vi "Create from SCP Send.vi"(4 "Permissions":T1={"Owner"={"Read"=TRUE, "Write"=TRUE, "Execute"=FALSE}, "Group"={"Read"=TRUE, "Write"=FALSE, "Execute"=FALSE}, "Others"={"Read"=TRUE, "Write"=FALSE, "Execute"=FALSE}}, 8 "Error In":errorcluster, 9 "File Size":i64, 10 "Remote Destination Path":string, 11 "Session":refnum<class "Session.lvclass">) -> (0 "Error Out":errorcluster, 3 "Channel":refnum<class "Channel.lvclass">)   [LabVIEW 2018, in "Toolkit.lvlib" / "Channel.lvclass"]
uses:
  Channel.lvclass
  Session/Session.lvclass
  Type Definitions/Permissions.ctl
  Type Definitions/Modes.ctl
  Session/Session.lvclass/Session.ctl
  SSH/SSH.lvclass/SSH.ctl
  Channel.lvclass/Channel.ctl
  Toolkit.lvlib
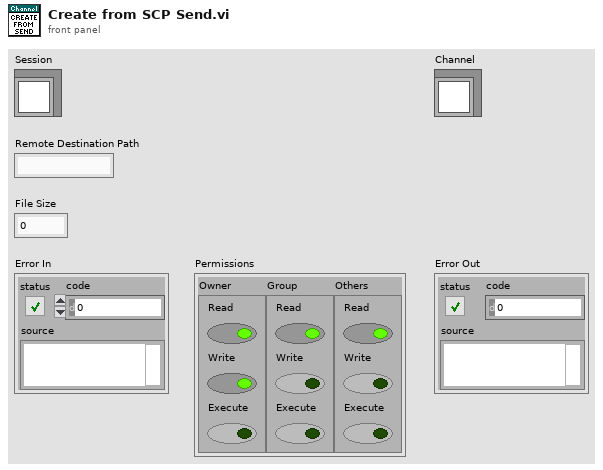
[diagram p1: front panel]
types:
  T1 = typedef "Toolkit.lvlib/Permissions.ctl" = cluster{"Owner":T2, "Group":T2, "Others":T2}
  T2 = typedef "Toolkit.lvlib/Modes.ctl" = cluster{"Read":bool, "Write":bool, "Execute":bool}
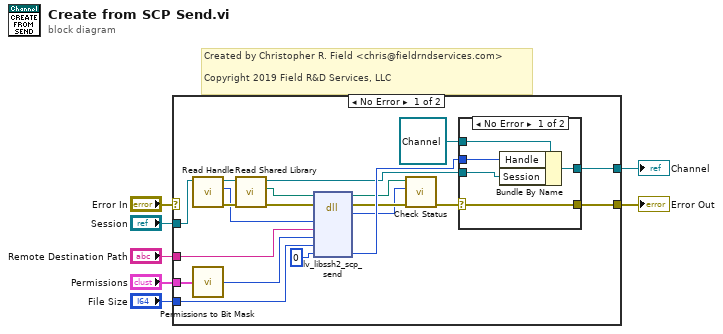
[diagram p0: block diagram]
diagram:
  # "Created by Christopher R. Field <chris@fieldrndservices.com>\n\nCopyright 2019 Field R&D Services, LLC"
  n1 = case shown="No Error" "Error In" {
    selector: "Error In" -> [_ w35]
    tunnel: [w25 w35] -> w6
    tunnel: "Session" -> [w26 _]
    tunnel: [w27 _] -> w4
    tunnel: "Permissions" -> [w23 _]
    tunnel: "Remote Destination Path" -> [w9 _]
    tunnel: "File Size" -> [w8 _]
    frame No Error {
      n2 = call "Read Handle.vi"("Session In"=w26) -> ("Erorr Out"=w21:errorcluster, "Handle"=w18:u64, "Session Out"=w22:refnum<class "Session.lvclass">)  [unwired: 8 in]
      n3 = call "Permissions to Bit Mask.vi"("Permissions"=w23) -> ("Bit Mask"=w10:u32)
      n4 = call "Read Shared Library.vi"("Error In"=w21, "Session In"=w22) -> ("Erorr Out"=w20:errorcluster, "libssh2lv Shared Library"=w19:path, "Session Out"=w11:refnum<class "Session.lvclass">)  [unwired: 7 in]
      n5 = dll-call lib="libssh2lv.*" fn="lv_libssh2_scp_send"(path in=w19, error in=w20, "session"=w18, "path"=w9, "mode"=w10, "file_size"=w8, "handle"=u64 0) -> (path out=w13:path, error out=w15:errorcluster, "status"=w14:i32, "handle"=w16:u64)  [unwired: 5 in]
      n6 = call "Check Status.vi"("Error In"=w15, "Status"=w14, "lv-libssh2 Shared Library In"=w13) -> ("Error Out"=w12:errorcluster)  [unwired: 7 in, 1 out]
      n7 = case shown="No Error" w12 {
        selector: w12 -> [w31 w34]
        tunnel: [w28 w33] -> w27
        tunnel: w16 -> [w32 _]
        tunnel: [w31 w34] -> w25
        tunnel: w11 -> [w30 _]
        tunnel: refnum<class "Channel.lvclass"> refnum ("Toolkit.lvlib:Channel.lvclass") -> [w29 w33]
        frame No Error {
          n8 = Bundle By Name(cluster=w29, "Handle"=w32, "Session"=w30) -> (w28:refnum<class "Channel.lvclass">)
        }
        frame Error {
        }
      }
    }
    frame Error {
    }
  }
  "Error Out" <- w6
  "Channel" <- w4
